vi "Motor.vi"(8 "INVERTI":bool, 10 "Fine":u16=4000, 11 "Change":i16) -> (1 "OutB":bool, 3 "outA":bool)   [LabVIEW 2017]
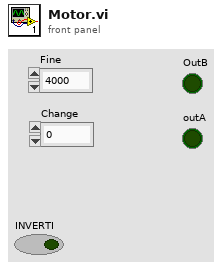
[diagram p1: front panel]
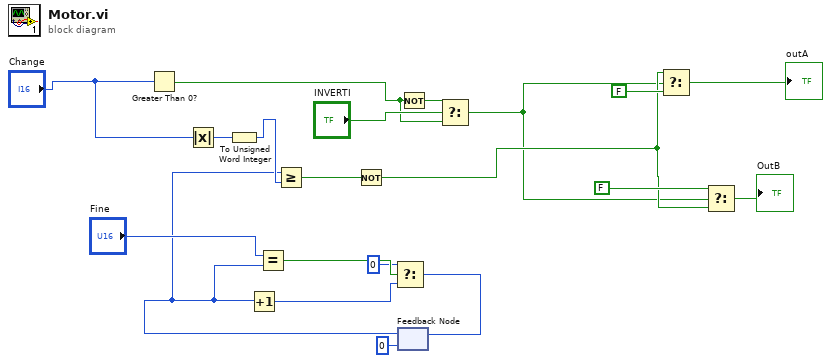
[diagram p0: block diagram]
diagram:
  n1 = Greater Than 0?(x="Change") -> (x > 0?=w2:bool)
  n2 = Absolute Value(x="Change") -> (abs(x)=w13:i16)
  n3 = To Unsigned Word Integer(number=w13) -> (unsigned 16bit integer=w12:u16)
  n4 = feedback #1(u16 0 ("t")) -> (w8:u16)
  n5 = Increment(x=w8) -> (x+1=w19:u16)
  n6 = Equal?(x="Fine", y=w8) -> (x = y?=w18:bool)
  n7 = Greater Or Equal?(x=w8, y=w12) -> (x >= y?=w5:bool)
  n8 = Not(x=w5) -> (.not. x?=w4:bool)
  n9 = Select(t=u16 0, s=w18, f=w19) -> (s? t:f=w9:u16)
  n10 = feedback-in #1(w9) -> ()
  n11 = Not(x=w2) -> (.not. x?=w3:bool)
  n12 = Select(t=w3, s="INVERTI", f=w2) -> (s? t:f=w1:bool)
  n13 = Select(t=w4, s=w1, f=FALSE) -> (s? t:f=→"outA":bool)
  n14 = Select(t=FALSE, s=w1, f=w4) -> (s? t:f=→"OutB":bool)
